vi "SendBulkMsg.vi"(7 "MsgType":T2=enum."DATA", 8 "error in":errorcluster, 10 "Payload":u16 format="%.0x", 11 "FPGA VI Reference In":T1) -> (0 "error out":errorcluster, 3 "FPGA VI Reference Out":T1)   [LabVIEW 2019]
uses:
  TypeDefs/Type of message.ctl
  TypeDefs/FPGA Reference.ctl
  <vilib>/Platform/TimedLoop/XDataNode/timing_clust.ctl
  <vilib>/Platform/TimedLoop/XDataNode/nitl_modes.ctl
  <vilib>/Platform/TimedLoop/XDataNode/wakeup.ctl
  <vilib>/Utility/error.llb/Error Cluster From Error Code.vi
  <vilib>/rvi/errors/niLvFpgaAdjustHostInterfaceError.vi
  <vilib>/Platform/TimedLoop/XDataNode/XDataNode.xnode
  <vilib>/rvi/interface/nirviMethod/nirviMethod.xnode
  FPGA Bitfiles/adafruitlcdsom_FPGATarget_FPGAMain_K7l+4zj6vFY.lvbitx
  FPGA Main.vi
  <vilib>/rvi/errors/niLvFpgaMergeErrorWithErrorCode.vi
  <vilib>/Platform/TimedLoop/XDataNode/XDNodeRunTimeDep.lvlib
  <vilib>/FPGAPlugInAG/sbRIO-9651/niLvFpga_WriteFifo_sbRIO-9651.vi
panel:
  in  "Loops":u32=19
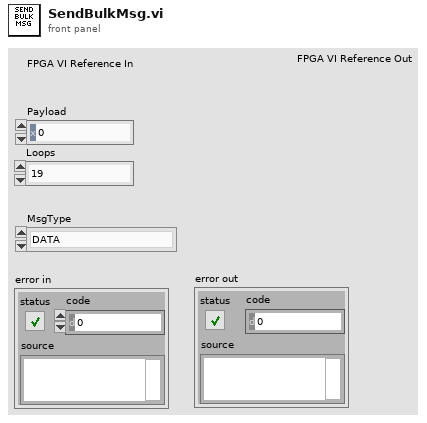
[diagram p1: front panel]
types:
  T1 = typedef "FPGA Reference.ctl" = refnum<k20>
  T2 = typedef "Type of message.ctl" = enum16{"CMD", "DATA"}
  T3 = typedef "XDNodeRunTimeDep.lvlib/timing_clust.ctl" = cluster{"Expected End [f-1]":u64, "Actual End [f-1]":u64, "Finished Late? [f-1]":bool, "Expected End [i-1]":u64, "Actual End [i-1]":u64, "Finished Late? [i-1]":bool, "Expected Start [i]":u64, "Actual Start [i]":u64, "Expected Start [f]":u64, "Actual Start [f]":u64, "Source Name":string, "Structure Name":string, "Period":i64, "Deadline":i64, "Offset":i64, "Start":i64, "Priority":i32, "Timeout":i32, "Mode":T4, "Wakeup Reason":T5, "Error":errorcluster, "Source Type":string, "Secondary Source Type":string, "Global End Time":u64, "Global Start Time":u64, "Frame Duration":u64, "Iteration Duration":u64, "Assigned CPU":i32, "I/O Scan Engine Mode":u32}
  T4 = typedef "XDNodeRunTimeDep.lvlib/nitl_modes.ctl" = enum32{"No Change", "Process missed periods, maintain original phase", "Discard missed periods, maintain original phase", "Process missed periods, ignore original phase", "Discard missed periods, ignore original phase"}
  T5 = typedef "XDNodeRunTimeDep.lvlib/wakeup.ctl" = enum32{"Normal", "Aborted", "Asynchronous wakeup", "Timing source error", "Timed loop error", "Timeout"}
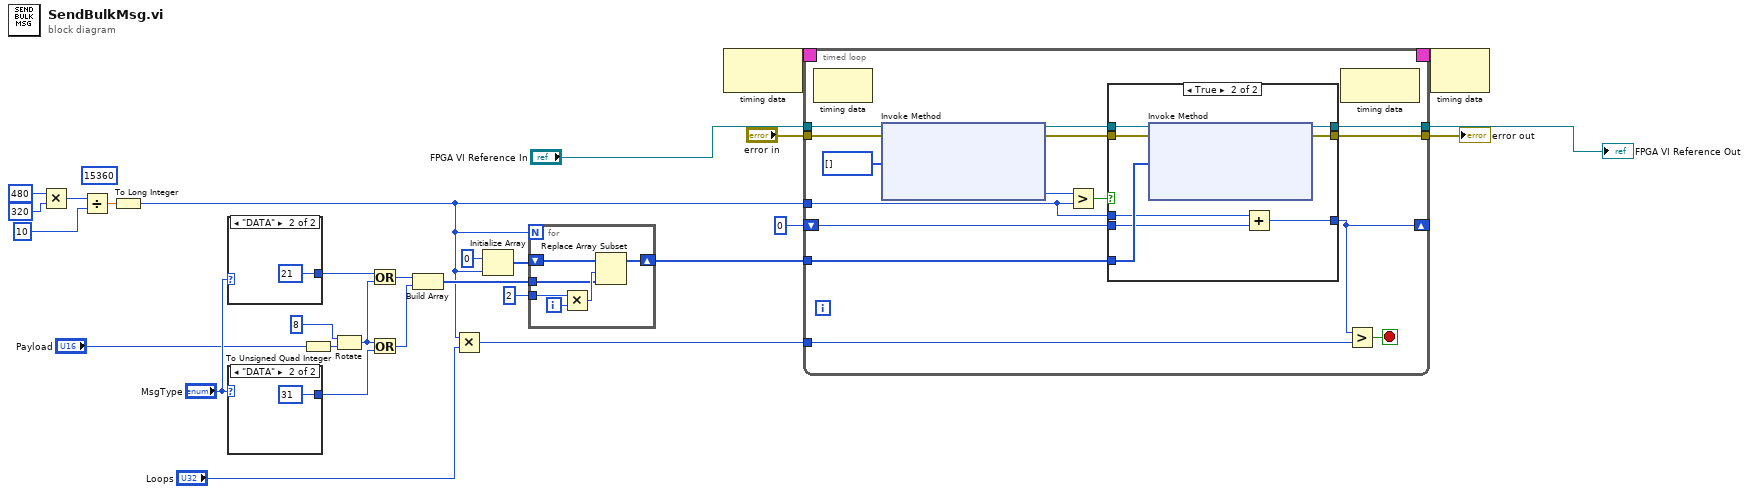
[diagram p0: block diagram]
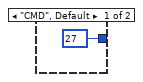
[diagram p3: hidden frame]
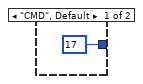
[diagram p4: hidden frame]
diagram:
  (unwired) u32 15360 ("dimension size")
  n1 = Multiply(x=480 ("dimension size"), y=320 ("dimension size")) -> (x*y=w9:i32)
  n2 = Divide(x=w9, y=10) -> (x/y=w7:dbl)
  n3 = To Long Integer(number=w7) -> (32bit integer=w4:i32)
  n4 = case shown="\"DATA\"" "MsgType" {
    tunnel: [u64 17 ("element") u64 21 ("element")] -> w28
    frame "CMD", Default {
    }
    frame "DATA" {
    }
  }
  n5 = case shown="\"DATA\"" "MsgType" {
    tunnel: [u64 27 ("element") u64 31 ("element")] -> w26
    frame "CMD", Default {
    }
    frame "DATA" {
    }
  }
  n6 = To Unsigned Quad Integer(1:"Payload") -> (0:w25:u64)
  n7 = Rotate(1:w25, 2:i16 8 ("y")) -> (0:w24:u64)
  n8 = Or(x=w28, y=w24) -> (x .or. y?=w27:u64)
  n9 = Or(x=w24, y=w26) -> (x .or. y?=w22:u64)
  n10 = Build Array(w27, w22) -> (w20:u64[])
  n11 = Multiply(x=w4, y="Loops") -> (x*y=w15:u32)
  n12 = Initialize Array(u64 0 ("element"), w4) -> (w18:u64[])
  n13 = for {
    N: w4 -> [_]
    tunnel: w20 -> [w36]
    shift-right: [w35] -> w5
    shift-left: w18 -> [w39]
    tunnel: 2 ("x") -> [w34]
    i -> [w38]
    n14 = Multiply(x=w34, y=w38) -> (x*y=w37:i32)
    n15 = Replace Array Subset(array=w39, new element=w36, index=w37) -> (w35:u64[])
  }
  n16 = node-c288() -> (w13:T3)  [unwired: 1 in]
  n17 = timed-loop {
    tunnel: "FPGA VI Reference In" -> [w53]
    tunnel: "error in" -> [w52]
    tunnel: w5 -> [w54]
    tunnel: w4 -> [w45]
    tunnel: [w47] -> w17
    tunnel: [w46] -> w1
    shift-right: [w43] -> _
    shift-left: u64 0 -> [w44]
    tunnel: w15 -> [w41]
    timing: w13 -> [_]
    timing-out: [_] -> w12
    stop <- w42 stop-if-true
    n18 = node-c288() -> ()  [unwired: 1 in, 1 out]
    n19 = xnode "Invoke Method"("FPGA VI Reference In"=w53, "error in"=w52, "Data"=u64[] []) -> ("FPGA VI Reference Out"=w50:T1, "error out"=w51:errorcluster, "Empty Elements Remaining"=w40:u32)  [unwired: 1 in]
    n20 = Greater?(x=w40, y=w45) -> (0:w48:bool)
    n21 = case shown="True" w48 {
      tunnel: w54 -> [_ w67]
      tunnel: w51 -> [w59 w66]
      tunnel: w50 -> [w58 w65]
      tunnel: [w59 w64] -> w47
      tunnel: [w58 w63] -> w46
      tunnel: w45 -> [_ w62]
      tunnel: [w57 w61] -> w43
      tunnel: w44 -> [w57 w60]
      frame False {
      }
      frame True {
        n22 = xnode "Invoke Method"("FPGA VI Reference In"=w65, "error in"=w66, "Data"=w67) -> ("FPGA VI Reference Out"=w63:T1, "error out"=w64:errorcluster)  [unwired: 1 in, 1 out]
        n23 = Add(x=w62, y=w60) -> (x+y=w61:u64)
      }
    }
    n24 = node-c288() -> ()  [unwired: 1 in, 1 out]
    n25 = Greater?(x=w43, y=w41) -> (0:w42:bool)
  }
  "error out" <- w17
  "FPGA VI Reference Out" <- w1
  n26 = node-c288(w12) -> ()  [unwired: 1 out]
